vi "encodeTimestamp.vi"(3 "Time Stamp":timestamp=timestamp(2082862800 s since 1904-01-01) format="%<%H:%M:%S%9u\n%x>T") -> (1 "MessagePack":u8[](array[numeric]) format="%.0x")   [LabVIEW 2015, in "MsgPack.lvlib"]
uses:
  MsgPack.lvlib
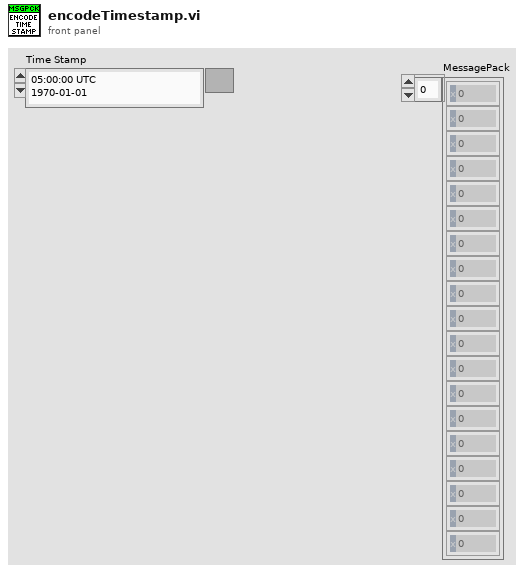
[diagram p1: front panel]
types:
  T1 = typedef "LVDateTimeRec.ctl" = cluster{"fractional second":dbl, "second":i32, "minute":i32, "hour":i32, "day of month":i32, "month":i32, "year":i32, "day of week":i32, "day of year":i32, "DST":i32}
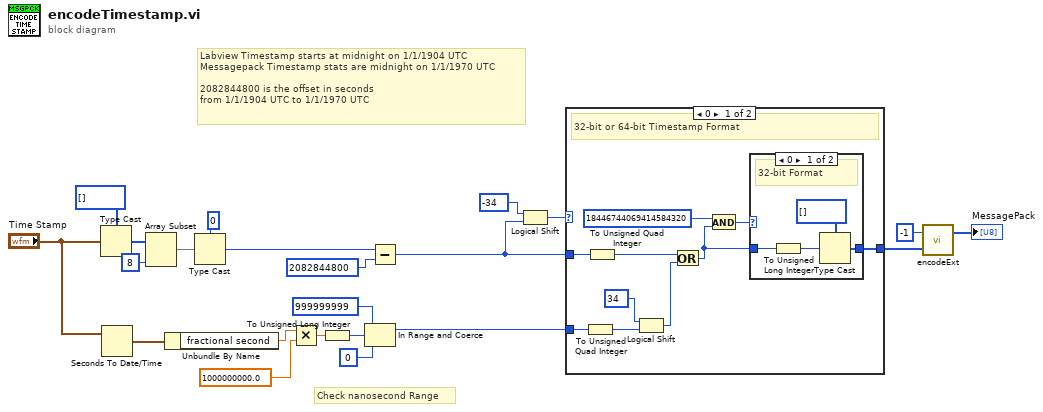
[diagram p0: block diagram]
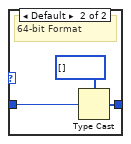
[diagram p2: hidden frame]
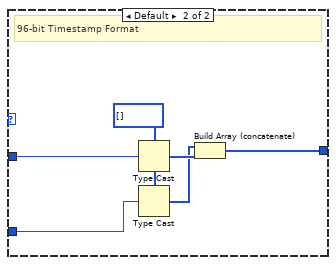
[diagram p3: hidden frame]
diagram:
  # "Check nanosecond Range"
  # "Labview Timestamp starts at midnight on 1/1/1904 UTC\nMessagepack Timestamp stats are midnight on 1/1/1970 UTC\n\n2082844800 is the offset in seconds\nfrom 1/1/1904 UTC to 1/1/1970 UTC"
  n1 = Type Cast(type=u8[] [] ("appended array"), x="Time Stamp") -> (*(type *) &x=w18:u8[])
  n2 = Seconds To Date/Time(time stamp (now)="Time Stamp") -> (date time rec=w20:T1)  [unwired: 1 in]
  n3 = Array Subset(array=w18, length=8) -> (w17:u8[])  [unwired: 1 in]
  n4 = Unbundle By Name(w20) -> ("fractional second"=w2:dbl)
  n5 = Type Cast(type=i64 0, x=w17) -> (*(type *) &x=w10:i64)
  n6 = Multiply(x=w2, y=1000000000.0) -> (x*y=w13:dbl)
  n7 = To Unsigned Long Integer(number=w13) -> (unsigned 32bit integer=w15:u32)
  n8 = In Range and Coerce(upper limit=u32 999999999, x=w15, lower limit=u32 0) -> (coerced(x)=w8:u32)  [unwired: 1 out]
  n9 = Subtract(x=w10, y=i64 2082844800) -> (x-y=w7:i64)
  n10 = Logical Shift(y=i64 -34 ("x"), x=w7) -> (x << y=w9:i64)
  n11 = case shown="0" w9 {
    tunnel: w7 -> [w31 w42]
    tunnel: w8 -> [w30 w41]
    tunnel: [w32 w40] -> w5
    frame 0 {
      # "32-bit or 64-bit Timestamp Format"
      n12 = To Unsigned Quad Integer(1:w30) -> (0:w24:u64)
      n13 = To Unsigned Quad Integer(1:w31) -> (0:w29:u64)
      n14 = Logical Shift(y=u64 34 ("x"), x=w24) -> (x << y=w28:u64)
      n15 = Or(x=w29, y=w28) -> (x .or. y?=w25:u64)
      n16 = And(x=u64 18446744069414584320 ("y"), y=w25) -> (x .and. y?=w26:u64)
      n17 = case shown="0" w26 {
        tunnel: [w33 w37] -> w32
        tunnel: w25 -> [w35 w38]
        frame 0 {
          # "32-bit Format"
          n18 = To Unsigned Long Integer(number=w35) -> (unsigned 32bit integer=w34:u32)
          n19 = Type Cast(type=u8[] [] ("appended array"), x=w34) -> (*(type *) &x=w33:u8[])
        }
        frame Default {
          # "64-bit Format"
          n20 = Type Cast(type=u8[] [] ("appended array"), x=w38) -> (*(type *) &x=w37:u8[])
        }
      }
    }
    frame Default {
      w44 = u8[] [] ("appended array")
      # "96-bit Timestamp Format"
      n21 = Type Cast(type=w44, x=w42) -> (*(type *) &x=w45:u8[])
      n22 = Type Cast(type=w44, x=w41) -> (*(type *) &x=w43:u8[])
      n23 = Build Array (concatenate)(w43, w45) -> (w40:u8[])
    }
  }
  n24 = call "encodeExt.vi"("ByteArray"=w5, "Type"=i8 -1) -> ("MessagePack"=→"MessagePack":u8[])  [unwired: 1 in]
